vi "Off.vi"(8 "error in (no error)":errorcluster, 11 "ThAr in":refnum<class "ThAr.lvclass">) -> (0 "error out":errorcluster, 3 "ThAr out":refnum<class "ThAr.lvclass">)   [LabVIEW 2016, in "ThAr.lvclass"]
uses:
  ThAr.lvclass
  Lamp.lvclass
panel:
  out "concatenated string":string
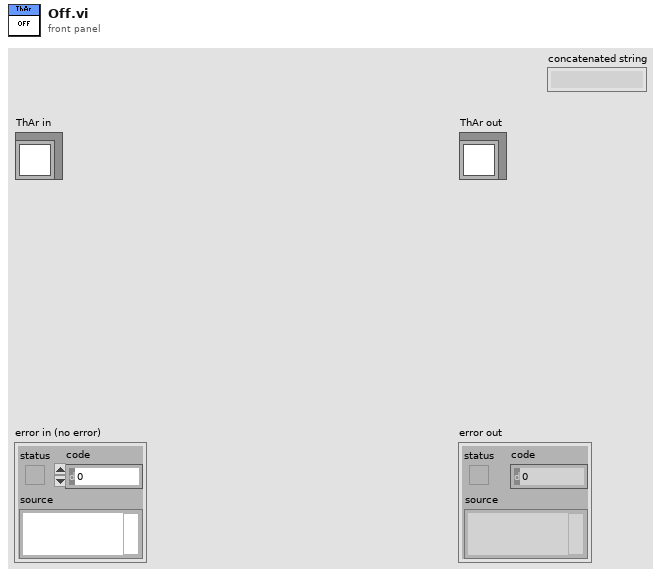
[diagram p1: front panel]
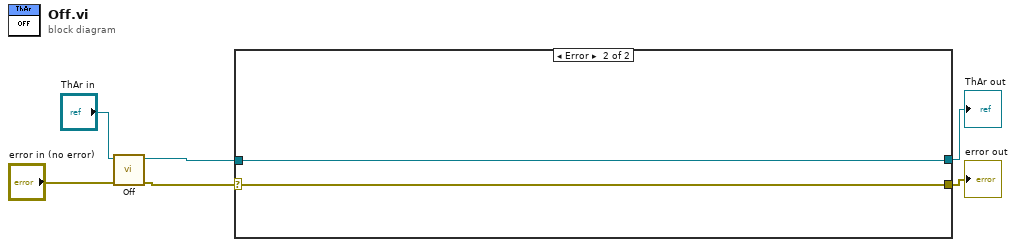
[diagram p0: block diagram]
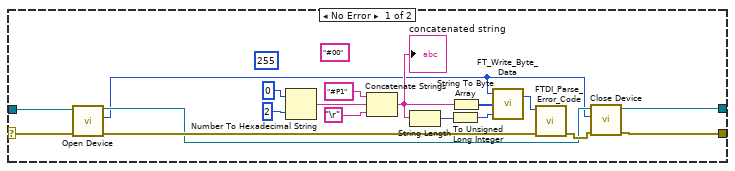
[diagram p2: hidden frame]
diagram:
  n1 = call-parent "Off.vi"("error in (no error)"="error in (no error)", "Lamp in"="ThAr in") -> ("error out"=w4:errorcluster, "Lamp out"=w3:refnum<class "ThAr.lvclass">)  [unwired: 8 in]
  n2 = case shown="Error" w4 {
    selector: w4 -> [w14 w26]
    tunnel: [w11 w26] -> w2
    tunnel: w3 -> [w12 w25]
    tunnel: [w7 w25] -> w1
    frame No Error {
      (unwired) 255 ("number")
      (unwired) "#00" ("Substring")
      n3 = call "Open Device.vi"("error in (no error)"=w14, "ThAr in"=w12) -> ("error constant"=w13:errorcluster, "Handle"=w8:u32, "ThAr out"=w9:refnum<class "ThAr.lvclass">)  [unwired: 7 in]
      n4 = Number To Hexadecimal String(1:i16 2 ("width (-)"), 2:0 ("number")) -> (0:w23:string)
      n5 = Concatenate Strings("#P1" ("Substring"), w23, "\r") -> (w18:string)
      "concatenated string" <- w18
      n6 = String Length(string=w18) -> (length=w21:i32)
      n7 = To Unsigned Long Integer(number=w21) -> (unsigned 32bit integer=w20:u32)
      n8 = String To Byte Array(string=w18) -> (unsigned byte array=w19:u8[])
      n9 = call "FT_Write_Byte_Data.vi"("Bytes To Write"=w20, "Buffer"=w19, "Handle"=w8) -> ("FT_Status"=w15:u32)  [unwired: 1 out]
      n10 = call "FTDI_Parse_Error_Code.vi"("error in (no error)"=w13, "FT_Status"=w15) -> ("error out"=w10:errorcluster)  [unwired: 9 in]
      n11 = call "Close Device.vi"("error in (no error)"=w10, "Handle"=w8, "ThAr in"=w9) -> ("error out"=w11:errorcluster, "ThAr out"=w7:refnum<class "ThAr.lvclass">)  [unwired: 7 in]
    }
    frame Error {
    }
  }
  "error out" <- w2
  "ThAr out" <- w1
